vi "DAQNavi Write (Analog 1D DBL 1Chan NSamp).vi"(8 "error in (no error)":errorcluster, 9 "timeout":dbl=10.0, 10 "data":dbl[](array[numeric]), 11 "task in":i32) -> (0 "error out":errorcluster, 2 "number of samples written per channel":u32, 3 "task out":i32)   [LabVIEW 2020]
uses:
  DAQNavi_LV.dll
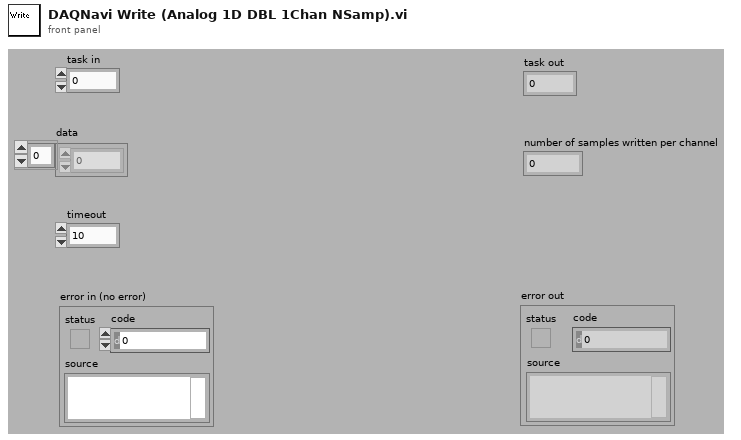
[diagram p1: front panel]
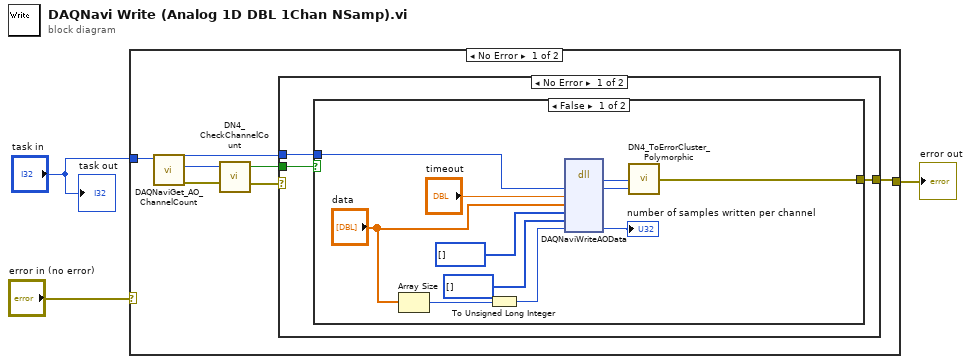
[diagram p0: block diagram]
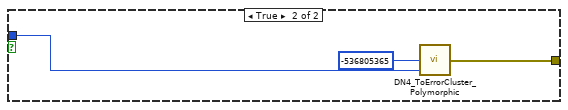
[diagram p2: hidden frame]
diagram:
  n1 = case shown="No Error" "error in (no error)" {
    selector: "error in (no error)" -> [_ w29]
    tunnel: [w9 w29] -> w2
    tunnel: "task in" -> [w10 _]
    frame No Error {
      n2 = call "DAQNaviGet_AO_ChannelCount.vi"("task in"=w10) -> ("error out"=w7:errorcluster, "channel count"=w8:i32, "task out"=w4:i32)  [unwired: 1 in, 7 out]
      n3 = call "DN4_CheckChannelCount.vi"("error out"=w7, "channel count"=w8) -> ("error IO"=w5:errorcluster, "greater than 1?"=w6:bool)  [unwired: 2 out]
      n4 = case shown="No Error" w5 {
        selector: w5 -> [_ w28]
        tunnel: w6 -> [w13 _]
        tunnel: w4 -> [w12 _]
        tunnel: [w11 w28] -> w9
        frame No Error {
          n5 = case shown="False" w13 {
            tunnel: [w18 w26] -> w11
            tunnel: w12 -> [w24 w25]
            frame False {
              n6 = Array Size(array="data") -> (size(s)=w16:i32)
              n7 = To Unsigned Long Integer(number=w16) -> (unsigned 32bit integer=w15:u32)
              n8 = dll-call lib="DAQNavi_LV.dll" fn="DAQNaviWriteAOData"("taskID"=w24, "timeout"="timeout", "scaledData"="data", "rawData16"=u16[] [], "rawData32"=u32[] [], "samples"=w15) -> ("return type"=w19:i32, "taskID"=w14:i32, "samples"=→"number of samples written per channel":u32)  [unwired: 5 in, 4 out]
              n9 = call "DN4_ToErrorCluster_Polymorphic.vi"("task id"=w14, "error code"=w19) -> ("error out"=w18:errorcluster)  [unwired: 3 out]
            }
            frame True {
              n10 = call "DN4_ToErrorCluster_Polymorphic.vi"("task id"=w25, "error code"=-536805365 ("error code (0)")) -> ("error out"=w26:errorcluster)  [unwired: 3 out]
            }
          }
        }
        frame Error {
        }
      }
    }
    frame Error {
    }
  }
  "error out" <- w2
  "task out" <- "task in"
